vi "prop_value_pair_main.vi"(10 "Value Pair Properties In":T1={"X Value Pairs"={"Data Array"=[], "Show ticks"=TRUE, "Show grid lines"=TRUE, "Labels"=enum."Name"}, "Y Value Pairs"={"Data Array"=[], "Show ticks"=TRUE, "Show grid lines"=TRUE, "Labels"=enum."Value"}, "Z Value Pairs"={"Data Array"=[], "Show ticks"=TRUE, "Show grid lines"=TRUE, "Labels"=enum."Value"}}) -> (2 "Value Pair Properties Out":T1={"X Value Pairs"={"Data Array"=[], "Show ticks"=TRUE, "Show grid lines"=TRUE, "Labels"=enum."Name"}, "Y Value Pairs"={"Data Array"=[], "Show ticks"=TRUE, "Show grid lines"=TRUE, "Labels"=enum."Value"}, "Z Value Pairs"={"Data Array"=[], "Show ticks"=TRUE, "Show grid lines"=TRUE, "Labels"=enum."Value"}})   [LabVIEW 2020, in "3DPC_SurfacePlot.xctl"]
uses:
  <vilib>/Native 3D Graph/xcontrol/3DPC_SurfacePlot.xctl
  <vilib>/Native 3D Graph/typedefs/prop_value_pair_all.ctl
  <vilib>/Native 3D Graph/typedefs/prop_value_pair_1d.ctl
  <vilib>/Utility/miscctls.llb/LVPointTypeDef.ctl
panel:
  in  "Axis Select":u16(ring) caption="Axis" items=["X", "Y", "Z"]
  in  "done":refnum<user-event>
  in  "quit":refnum<user-event>
  in  "Axes Control Tab":enum32{"X", "Y", "Z"}(tab)
  in  "Labels X":u16(ring) caption="Labels" items=["Value", "None", "Name"]
  in  "Show Ticks X":bool
  in  "Show Grid Lines X":bool
  in  "Delete X":bool
  in  "Add X":bool
  in  "Pair Table X":i32(listbox)
  in  "Name X":string caption="Name"
  in  "Value X":dbl caption="Value"
  in  "Labels Y":u16(ring) caption="Labels" items=["Value", "None", "Name"]
  in  "Show Ticks Y":bool
  in  "Show Grid Lines Y":bool
  in  "Pair Table Y":i32(listbox)
  in  "Name Y":string caption="Name"
  in  "Value Y":dbl caption="Value"
  in  "Add Y":bool
  in  "Delete Y":bool
  in  "Labels Z":u16(ring) caption="Labels" items=["Value", "None", "Name"]
  in  "Show Ticks Z":bool
  in  "Show Grid Lines Z":bool
  in  "Pair Table Z":i32(listbox)
  in  "Name Z":string caption="Name"
  in  "Value Z":dbl caption="Value"
  in  "Delete Z":bool
  in  "Add Z":bool
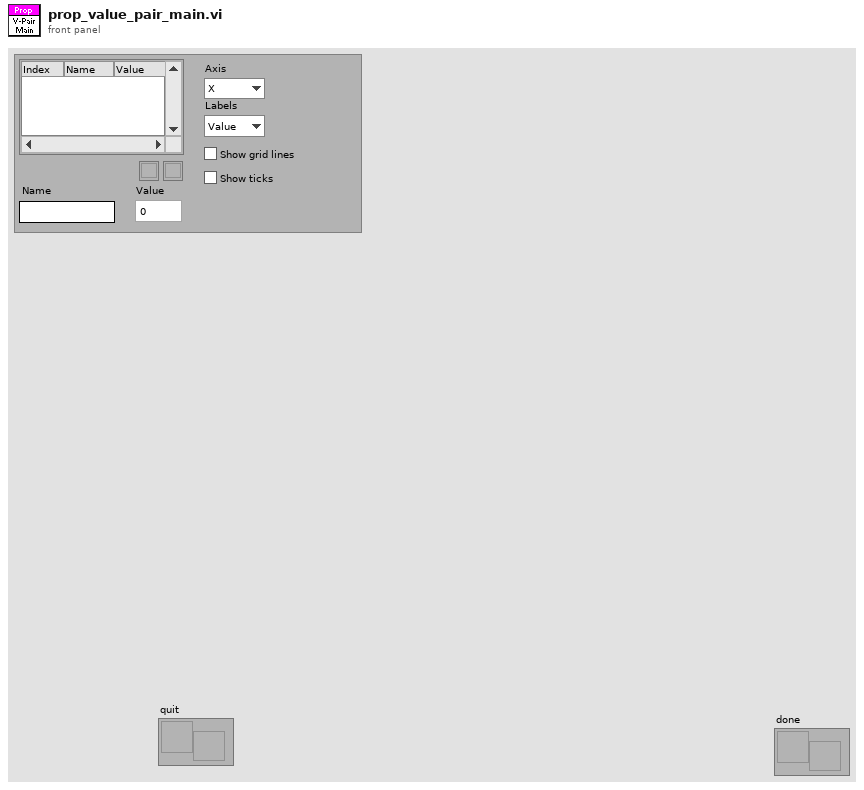
[diagram p1: front panel]
types:
  T1 = typedef "3DPC_SurfacePlot.xctl/prop_value_pair_all.ctl" = cluster{"X Value Pairs":cluster{"Data Array":cluster{"Value":sgl, "Index":i32, "Name":string}[], "Show ticks":bool, "Show grid lines":bool, "Labels":enum16{"Value", "None", "Name"}}, "Y Value Pairs":T2, "Z Value Pairs":T2}
  T2 = typedef "3DPC_SurfacePlot.xctl/prop_value_pair_1d.ctl" = cluster{"Data Array":cluster{"Value":sgl, "Index":i32, "Name":string}[], "Show ticks":bool, "Show grid lines":bool, "Labels":enum16{"Value", "None", "Name"}}
  T3 = typedef "LVPointTypeDef.ctl" = cluster{"Horizontal":i16, "Vertical":i16}
  T4 = cluster{"Value":sgl, "Index":i32, "Name":string}[]
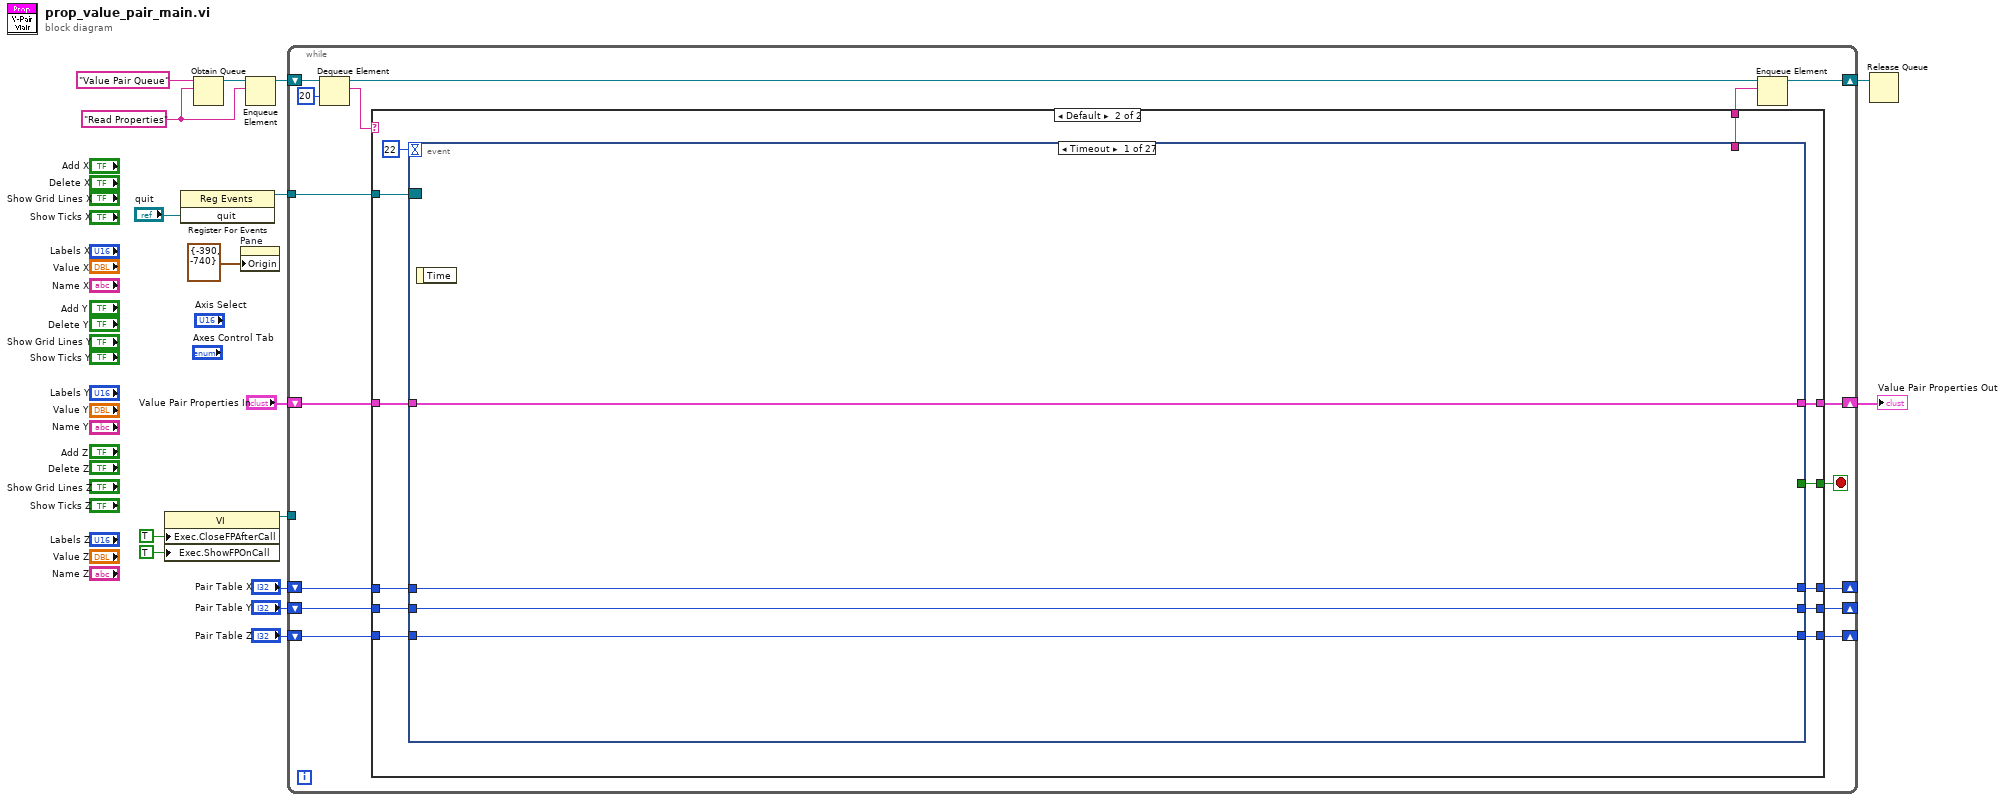
[diagram p0: block diagram]
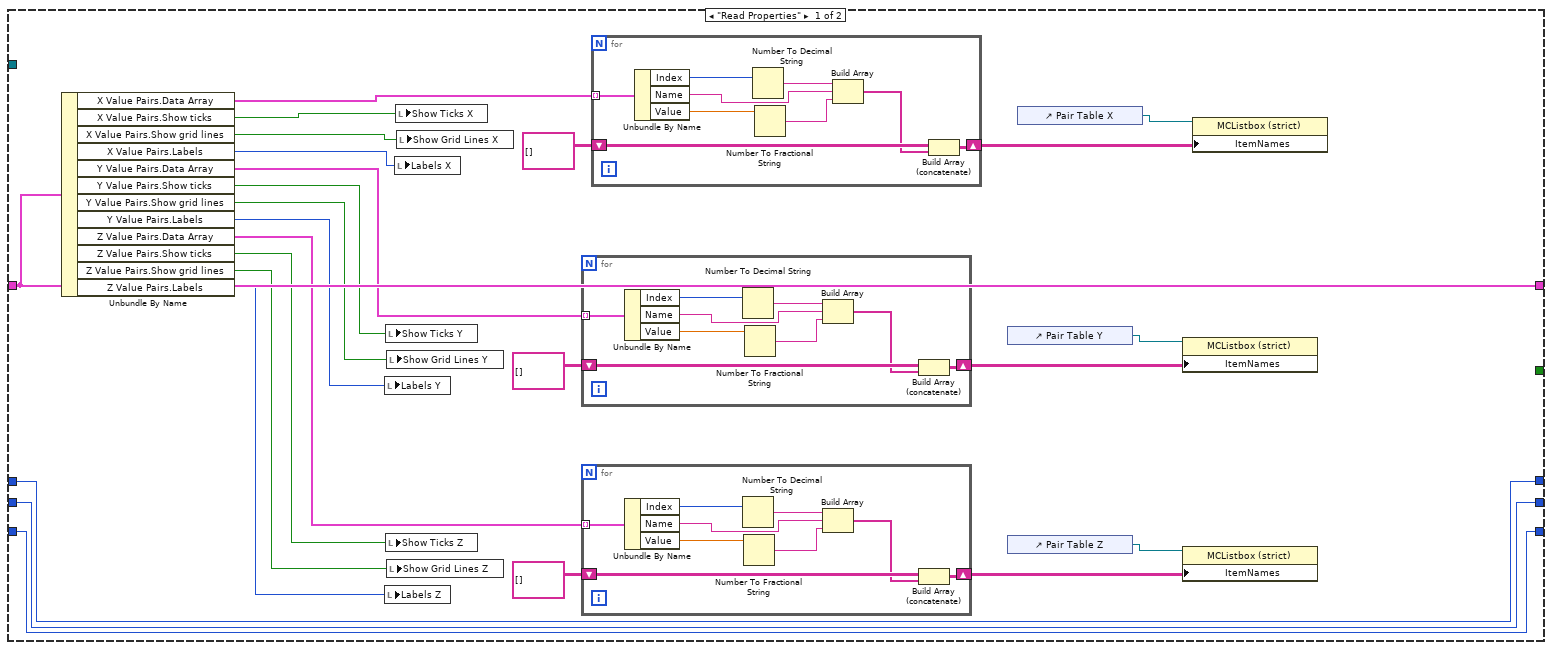
[diagram p2: hidden frame]
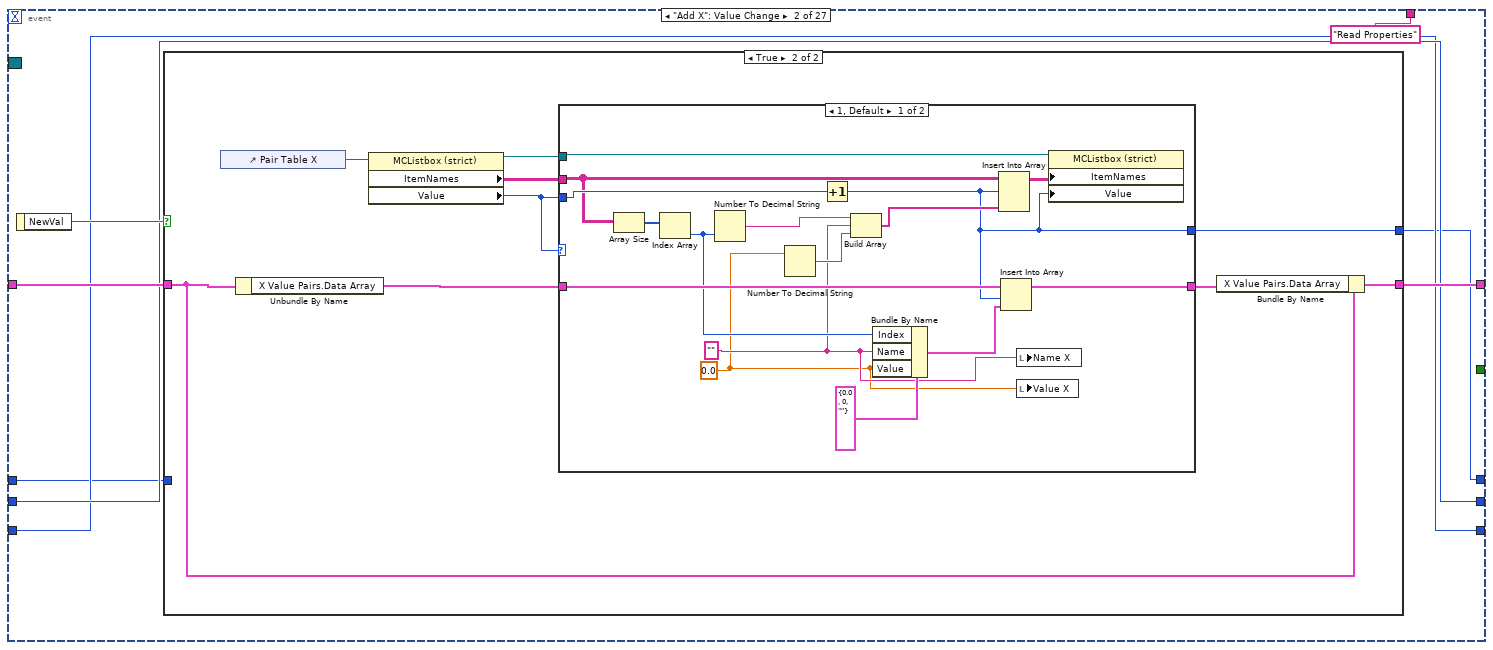
[diagram p3: hidden frame]
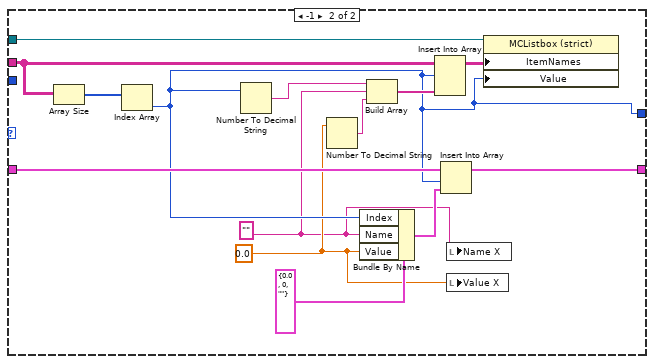
[diagram p5: hidden frame]
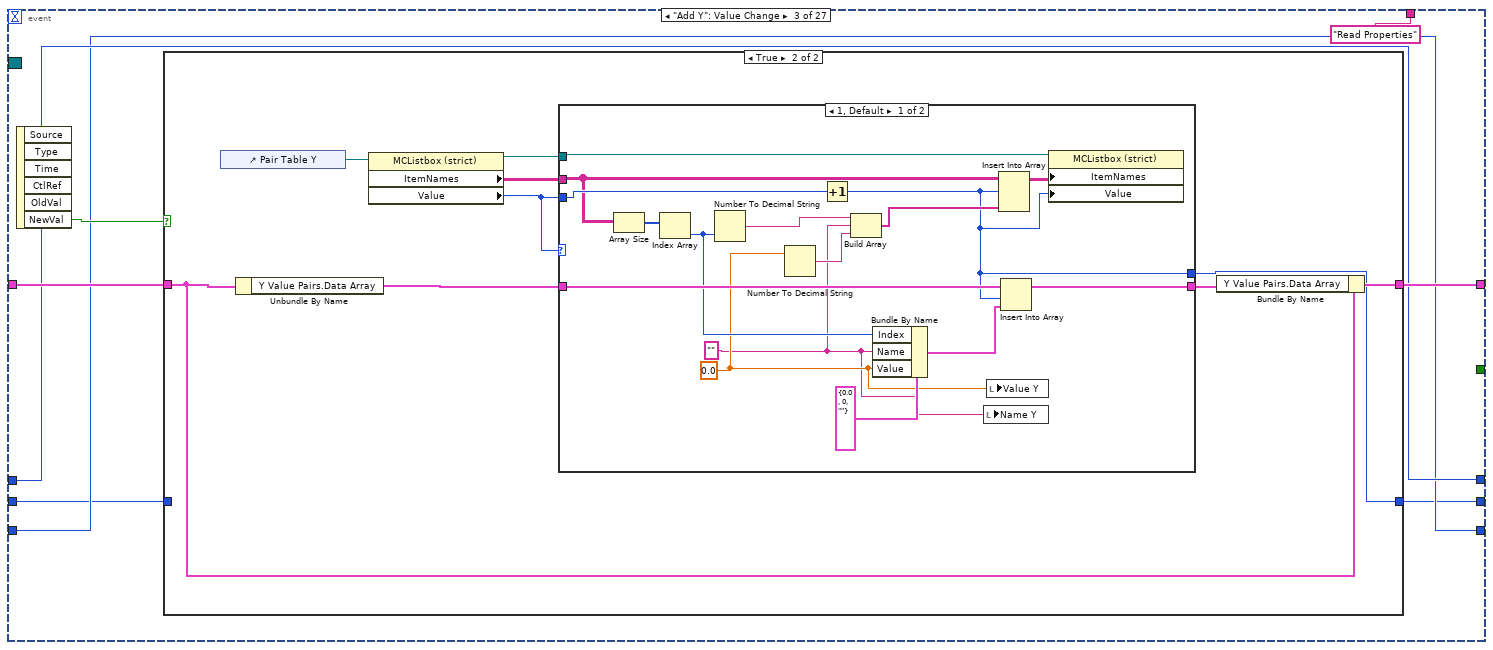
[diagram p6: hidden frame]
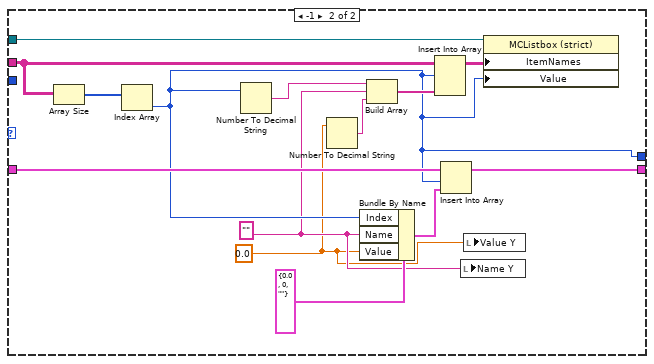
[diagram p8: hidden frame]
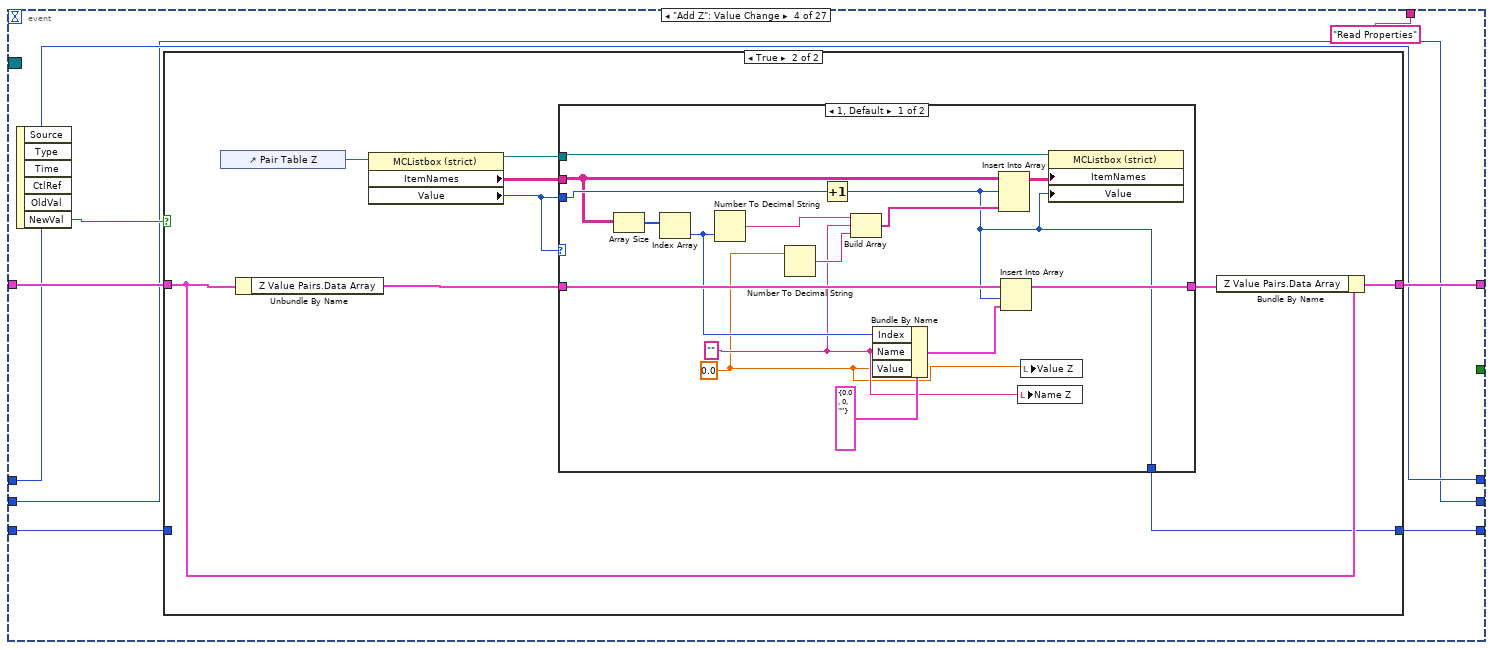
[diagram p9: hidden frame]
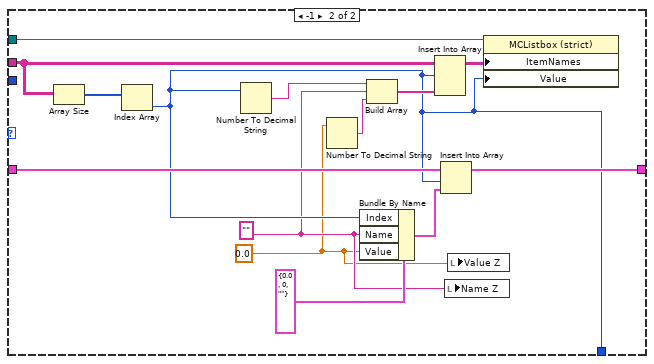
[diagram p11: hidden frame]
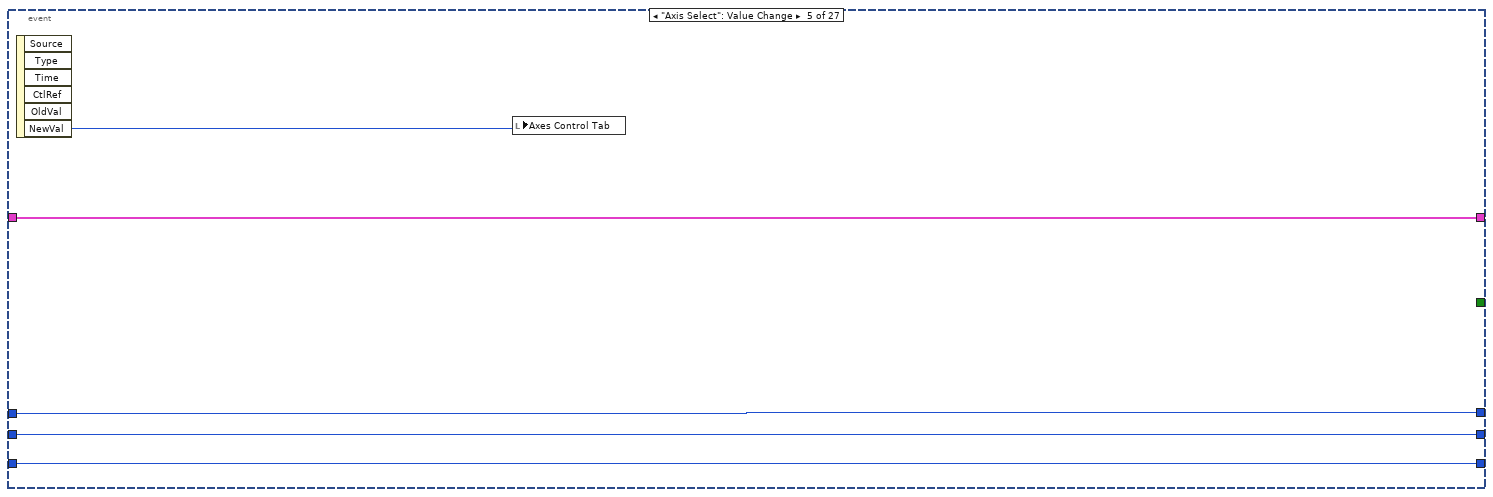
[diagram p12: hidden frame]
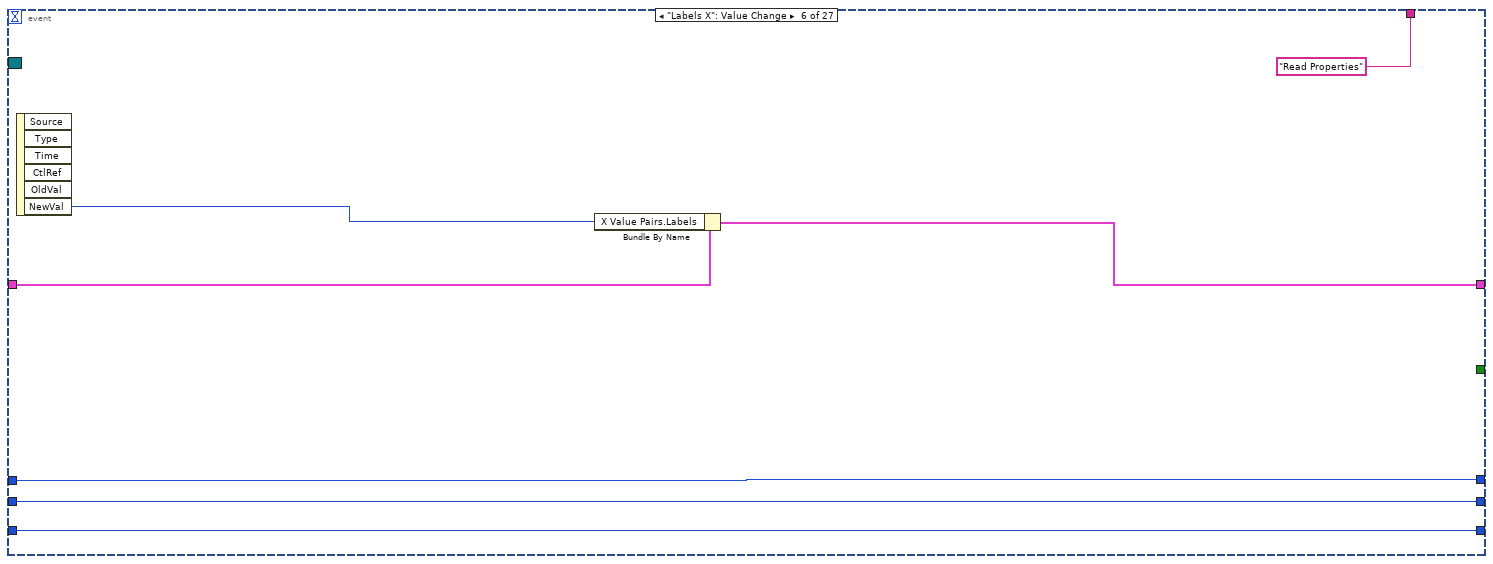
[diagram p13: hidden frame]
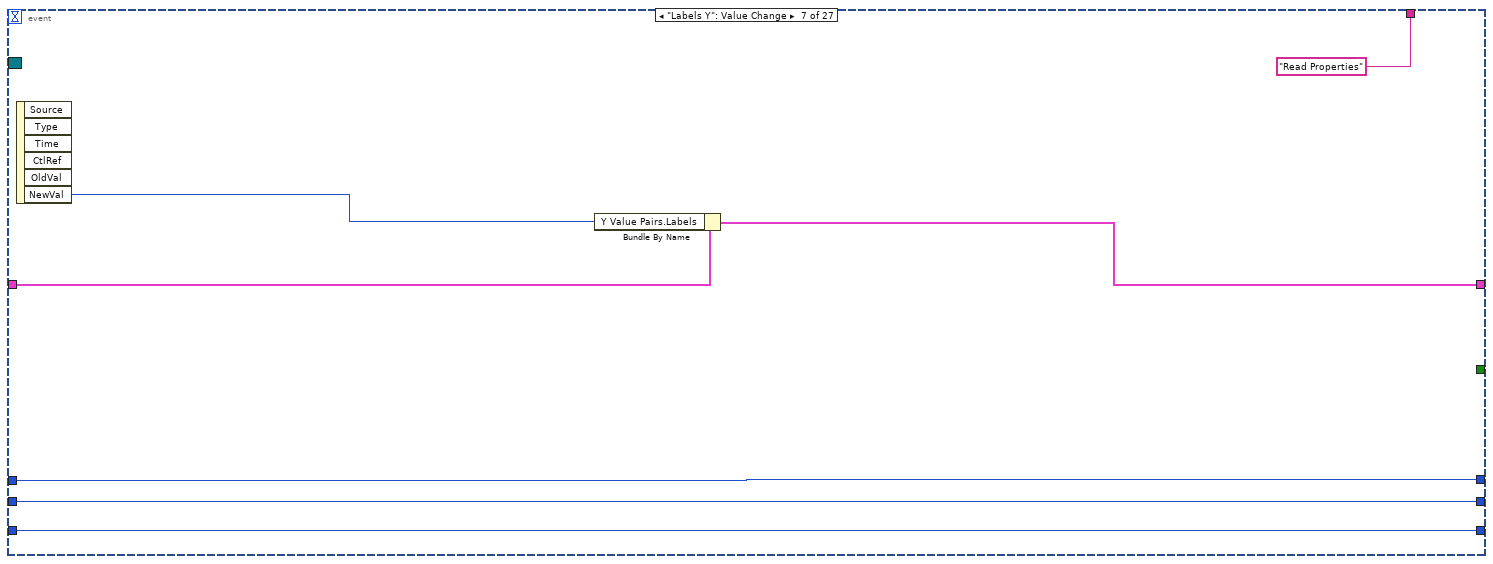
[diagram p14: hidden frame]
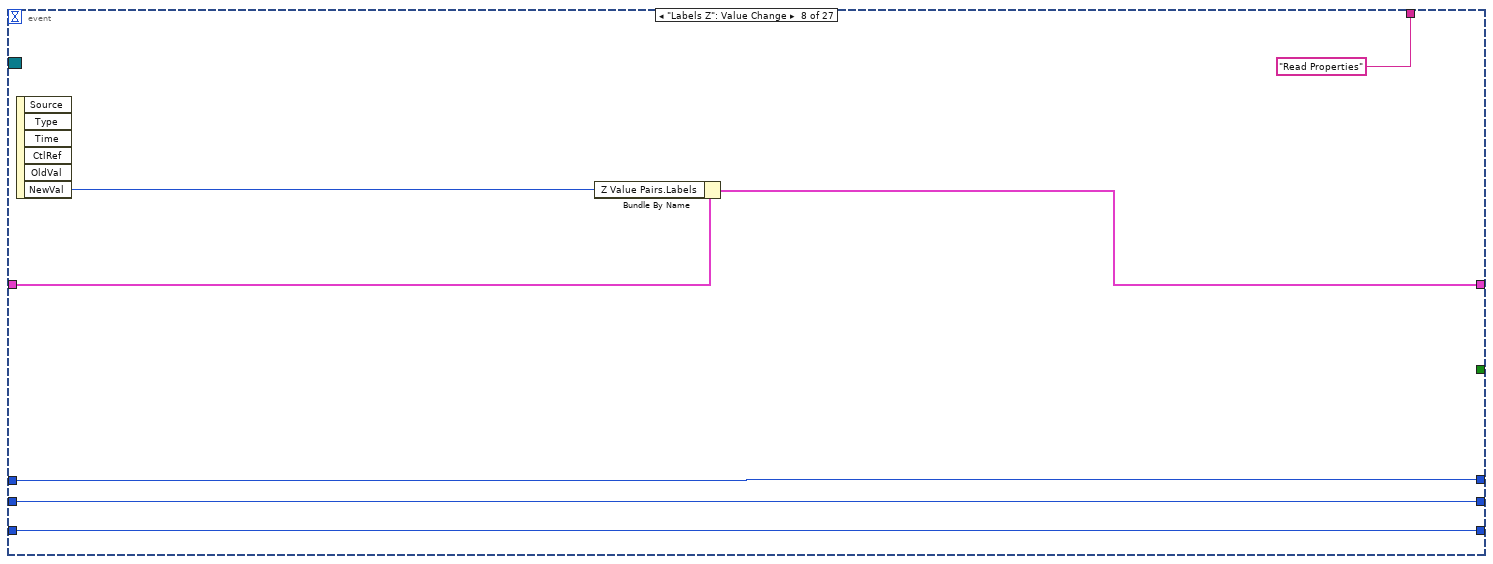
[diagram p15: hidden frame]
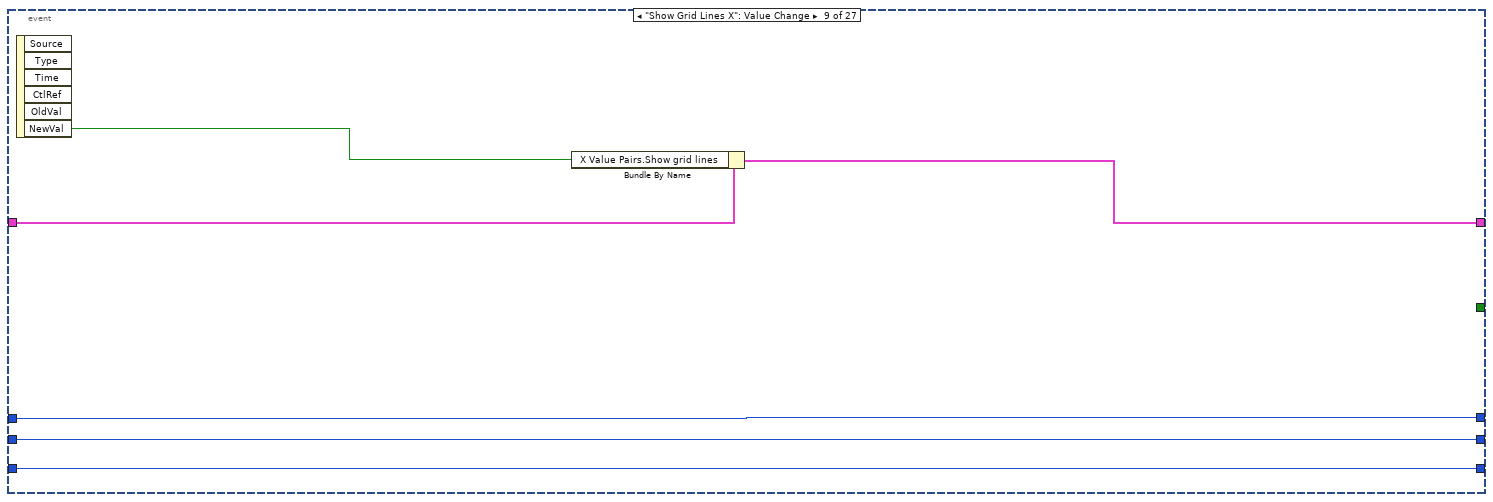
[diagram p16: hidden frame]
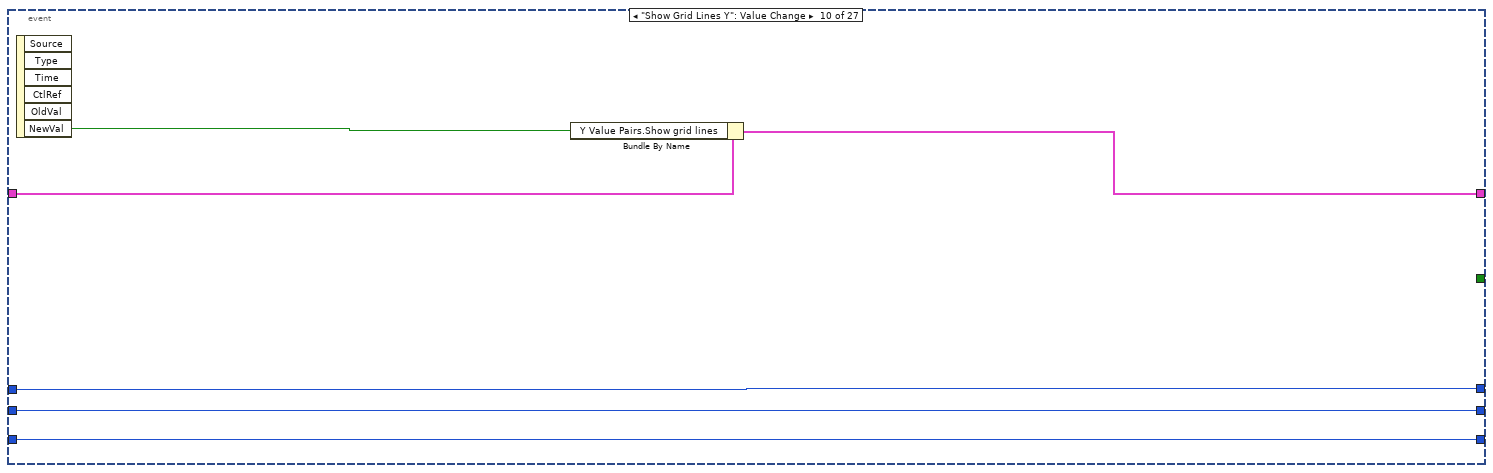
[diagram p17: hidden frame]
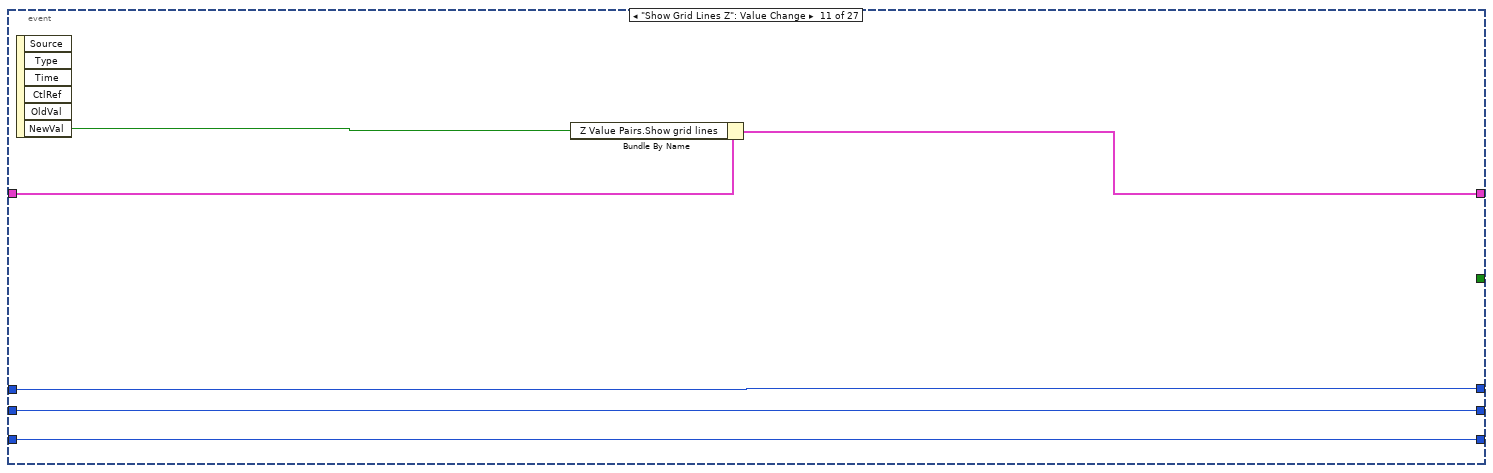
[diagram p18: hidden frame]
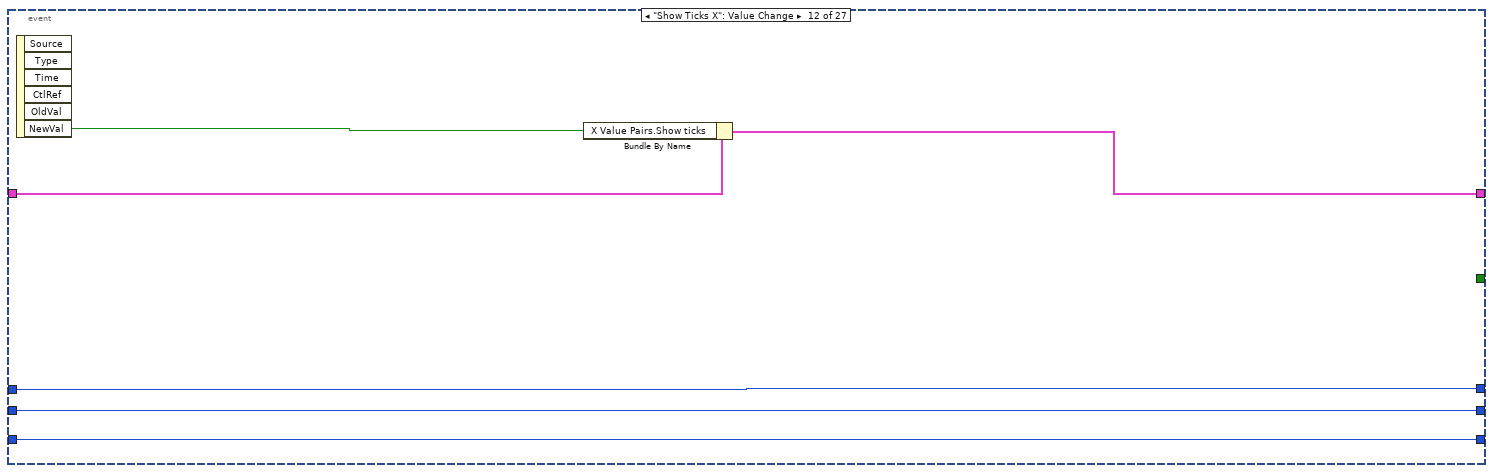
[diagram p19: hidden frame]
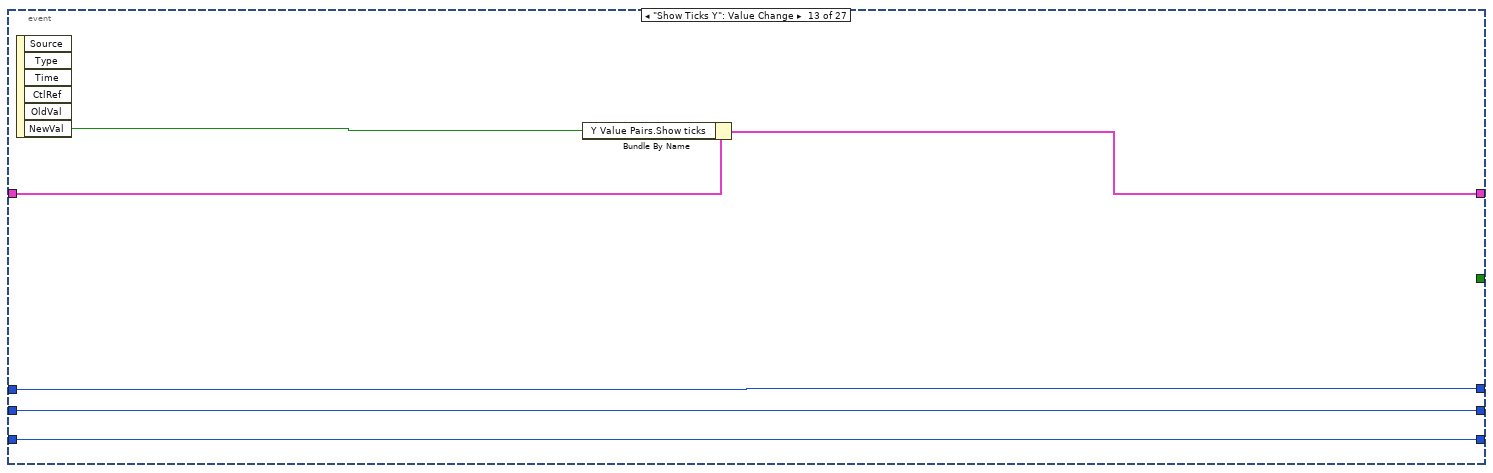
[diagram p20: hidden frame]
diagram:
  w13 = "Read Properties"
  n1 = property class="VI"("Exec.CloseFPAfterCall"=TRUE ("Execution:Close After Call"), "Exec.ShowFPOnCall"=TRUE ("Execution:Show Front Panel On Call")) -> (reference out=w10:refnum<vi>)  [unwired: 2 in, 1 out]
  n2 = register-events("quit") -> (reference out=w8:refnum<event-registration>)  [unwired: 2 in, 1 out]
  n3 = Obtain Queue(name (unnamed)="Value Pair Queue", element data type=w13) -> (queue out=w15:refnum<queue>)  [unwired: 3 in, 2 out]
  n4 = property on="Pane" class="Pane"("Origin"=T3 {"Horizontal"=-390, "Vertical"=-740}) -> ()  [unwired: 2 in, 2 out]
  n5 = Enqueue Element(queue=w15, element=w13) -> (queue out=w14:refnum<queue>)  [unwired: 1 in, 3 out]
  n6 = while {
    shift-right: [w29] -> w11
    shift-left: w14 -> [w32]
    shift-right: [w25] -> w12
    shift-left: "Value Pair Properties In" -> [w26]
    tunnel: w10 -> [_]
    tunnel: w8 -> [w23]
    shift-right: [w21] -> _
    shift-left: "Pair Table X" -> [w22]
    shift-right: [w20] -> _
    shift-left: "Pair Table Z" -> [w17]
    shift-right: [w19] -> _
    shift-left: "Pair Table Y" -> [w18]
    stop <- w24 stop-if-true
    n7 = Dequeue Element(queue=w32, timeout in ms (-1)=20) -> (queue out=w30:refnum<queue>, element=w31:string)  [unwired: 1 in, 2 out]
    n8 = case shown="Default" w31 {
      tunnel: [_ w95] -> w24
      tunnel: [_ w93] -> w28
      tunnel: w26 -> [w50 w96]
      tunnel: [w50 w94] -> w25
      tunnel: w23 -> [_ w91]
      tunnel: w22 -> [w35 w90]
      tunnel: w18 -> [w34 w89]
      tunnel: w17 -> [w33 w88]
      tunnel: [w35 w87] -> w21
      tunnel: [w33 w86] -> w20
      tunnel: [w34 w85] -> w19
      frame "Read Properties" {
        n9 = Unbundle By Name(w50) -> ("X Value Pairs.Data Array"=w57:T4, "X Value Pairs.Show ticks"=w55:bool, "X Value Pairs.Show grid lines"=w54:bool, "X Value Pairs.Labels"=w53:enum16{"Value", "None", "Name"}, "Y Value Pairs.Data Array"=w43:T4, "Y Value Pairs.Show ticks"=w42:bool, "Y Value Pairs.Show grid lines"=w41:bool, "Y Value Pairs.Labels"=w40:enum16{"Value", "None", "Name"}, "Z Value Pairs.Data Array"=w39:T4, "Z Value Pairs.Show ticks"=w38:bool, "Z Value Pairs.Show grid lines"=w37:bool, "Z Value Pairs.Labels"=w36:enum16{"Value", "None", "Name"})
        n10 = local write "Labels Y"(w40) -> ()
        n11 = local write "Labels Z"(w36) -> ()
        n12 = local write "Show Ticks Y"(w42) -> ()
        n13 = local write "Show Ticks Z"(w38) -> ()
        n14 = local write "Show Grid Lines Y"(w41) -> ()
        n15 = local write "Show Grid Lines Z"(w37) -> ()
        n16 = local write "Labels X"(w53) -> ()
        n17 = local write "Show Ticks X"(w55) -> ()
        n18 = local write "Show Grid Lines X"(w54) -> ()
        n19 = for {
          tunnel: w43 -> [w75] mode=indexing
          shift-right: [w70] -> w48
          shift-left: string[][] [] -> [w72]
          n20 = Unbundle By Name(w75) -> ("Index"=w74:i32, "Name"=w69:string, "Value"=w67:sgl)
          n21 = Number To Decimal String(number=w74) -> (decimal integer string=w73:string)  [unwired: 1 out]
          n22 = Number To Fractional String(number=w67) -> (F-format string=w68:string)  [unwired: 3 out]
          n23 = Build Array(w73, w69, w68) -> (w71:string[])
          n24 = Build Array (concatenate)(w72, w71) -> (w70:string[][])
        }
        n25 = for {
          tunnel: w39 -> [w66] mode=indexing
          shift-right: [w61] -> w45
          shift-left: string[][] [] -> [w63]
          n26 = Unbundle By Name(w66) -> ("Index"=w65:i32, "Name"=w60:string, "Value"=w58:sgl)
          n27 = Number To Decimal String(number=w65) -> (decimal integer string=w64:string)  [unwired: 1 out]
          n28 = Number To Fractional String(number=w58) -> (F-format string=w59:string)  [unwired: 3 out]
          n29 = Build Array(w64, w60, w59) -> (w62:string[])
          n30 = Build Array (concatenate)(w63, w62) -> (w61:string[][])
        }
        n31 = for {
          tunnel: w57 -> [w84] mode=indexing
          shift-right: [w79] -> w52
          shift-left: string[][] [] -> [w81]
          n32 = Unbundle By Name(w84) -> ("Index"=w83:i32, "Name"=w78:string, "Value"=w76:sgl)
          n33 = Number To Decimal String(number=w83) -> (decimal integer string=w82:string)  [unwired: 1 out]
          n34 = Number To Fractional String(number=w76) -> (F-format string=w77:string)  [unwired: 3 out]
          n35 = Build Array(w82, w78, w77) -> (w80:string[])
          n36 = Build Array (concatenate)(w81, w80) -> (w79:string[][])
        }
        n37 = control-ref of="Pair Table Y"() -> (w49:refnum<vi>)
        n38 = control-ref of="Pair Table Z"() -> (w44:refnum<vi>)
        n39 = control-ref of="Pair Table X"() -> (w51:refnum<vi>)
        n40 = property class="MCListbox (strict)"(reference=w49, "ItemNames"=w48) -> ()  [unwired: 1 in, 2 out]
        n41 = property class="MCListbox (strict)"(reference=w44, "ItemNames"=w45) -> ()  [unwired: 1 in, 2 out]
        n42 = property class="MCListbox (strict)"(reference=w51, "ItemNames"=w52) -> ()  [unwired: 1 in, 2 out]
      }
      frame Default {
        n43 = event shown="[0] Timeout" {
          selector: w91 -> [_ _ _ _ _ _ _ _ _ _ _ _ _ _ _ _ _ _ _ _ _ _ _ _ _ _ _]
          dyn-events: _ -> [_ _ _ _ _ _ _ _ _ _ _ _ _ _ _ _ _ _ _ _ _ _ _ _ _ _ _]
          timeout: 22 -> [_ _ _ _ _ _ _ _ _ _ _ _ _ _ _ _ _ _ _ _ _ _ _ _ _ _ _]
          tunnel: w96 -> [w100 w107 w156 w205 w251 w259 w266 w273 w279 w285 w291 w297 w303 w309 w317 w325 w333 w338 w354 w370 w392 w403 w414 w425 w432 w443 w455]
          tunnel: [_ _ _ _ _ _ _ _ _ _ _ _ _ _ _ _ _ _ _ _ _ _ _ _ TRUE _ FALSE ("NewVal")] -> w95
          tunnel: [w100 w106 w155 w204 w251 w257 w264 w271 w277 w283 w289 w295 w301 w307 w317 w325 w333 w337 w353 w369 w387 w398 w409 w420 w432 w438 w450] -> w94
          tunnel: [_ "Read Properties" "Read Properties" "Read Properties" _ "Read Properties" "Read Properties" "Read Properties" _ _ _ _ _ _ _ _ _ _ _ _ "Read Properties" "Read Properties" "Read Properties" "Read Properties" _ "Read Properties" "Read Properties"] -> w93
          tunnel: w90 -> [w99 w102 w154 w203 w250 w255 w262 w269 w276 w282 w288 w294 w300 w306 _ w318 w326 w334 w352 w366 w384 w395 w406 w417 w428 w433 w444]
          tunnel: w89 -> [w98 w105 w151 w202 w249 w254 w261 w268 w275 w281 w287 w293 w299 w305 w311 _ w327 w336 w350 w367 w383 w394 w405 w415 w427 w435 w445]
          tunnel: w88 -> [w97 w104 w153 w200 w248 w253 w260 w267 w274 w280 w286 w292 w298 w304 w310 w319 _ w335 w351 w368 w382 w393 w404 w416 w426 w434 w446]
          tunnel: [w99 w103 w154 w203 w250 w255 w262 w269 w276 w282 w288 w294 w300 w306 w312 w318 w326 w334 w352 w366 w384 w395 w406 w417 w428 w433 w444] -> w87
          tunnel: [w97 w104 w153 w201 w248 w253 w260 w267 w274 w280 w286 w292 w298 w304 w310 w319 w328 w335 w351 w368 w382 w393 w404 w416 w426 w434 w446] -> w86
          tunnel: [w98 w105 w152 w202 w249 w254 w261 w268 w275 w281 w287 w293 w299 w305 w311 w320 w327 w336 w350 w367 w383 w394 w405 w415 w427 w435 w445] -> w85
          event Timeout {
            n44 = event-data() -> ()  [unwired: 2 out]
          }
          event "Add X": Value Change {
            n45 = event-data() -> ("NewVal"=w108:bool)  [unwired: 1 out]
            n46 = case shown="True" w108 {
              tunnel: w107 -> [w110 w113]
              tunnel: [w110 w114] -> w106
              tunnel: [w109 w111] -> w103
              tunnel: w102 -> [w109 _]
              frame False {
              }
              frame True {
                n47 = control-ref of="Pair Table X"() -> (w119:refnum<vi>)
                n48 = Unbundle By Name(w113) -> ("X Value Pairs.Data Array"=w115:T4)
                n49 = property class="MCListbox (strict)"(reference=w119) -> (reference out=w118:refnum<vi>, "ItemNames"=w117:string[][], "Value"=w116:i32)  [unwired: 1 in, 1 out]
                n50 = case shown="1, Default" w116 {
                  tunnel: w118 -> [w135 w149]
                  tunnel: w117 -> [w130 w145]
                  tunnel: w116 -> [w131 _]
                  tunnel: w115 -> [w127 w140]
                  tunnel: [w123 w139] -> w112
                  tunnel: [w122 w138] -> w111
                  frame 1, Default {
                    w120 = sgl 0.0 ("Value")
                    w121 = "" ("decimal integer string")
                    n51 = Array Size(array=w130) -> (size(s)=w129:i32[])
                    n52 = Index Array(array=w129) -> (element=w125:i32)  [unwired: 1 in]
                    n53 = Number To Decimal String(number=w125) -> (decimal integer string=w132:string)  [unwired: 1 out]
                    n54 = Number To Decimal String(number=w120) -> (decimal integer string=w124:string)  [unwired: 1 out]
                    n55 = Increment(x=w131) -> (x+1=w122:i32)
                    n56 = Build Array(w132, w121, w124) -> (w133:string[])
                    n57 = Bundle By Name(cluster=cluster{"Value":sgl, "Index":i32, "Name":string} {"Value"=0.0, "Index"=0, "Name"=""}, "Index"=w125, "Name"=w121, "Value"=w120) -> (w126:cluster{"Value":sgl, "Index":i32, "Name":string})
                    n58 = Insert Into Array(array=w130, index (row)=w122, new element=w133) -> (w134:string[][])  [unwired: 1 in]
                    n59 = Insert Into Array(array=w127, index=w122, new element=w126) -> (w123:T4)
                    n60 = local write "Name X"(w121) -> ()
                    n61 = local write "Value X"(w120) -> ()
                    n62 = property class="MCListbox (strict)"(reference=w135, "ItemNames"=w134, "Value"=w122) -> ()  [unwired: 1 in, 2 out]
                  }
                  frame -1 {
                    w137 = sgl 0.0 ("Value")
                    w136 = "" ("decimal integer string")
                    n63 = Array Size(array=w145) -> (size(s)=w144:i32[])
                    n64 = Index Array(array=w144) -> (element=w138:i32)  [unwired: 1 in]
                    n65 = Number To Decimal String(number=w138) -> (decimal integer string=w146:string)  [unwired: 1 out]
                    n66 = Number To Decimal String(number=w137) -> (decimal integer string=w141:string)  [unwired: 1 out]
                    n67 = Bundle By Name(cluster=cluster{"Value":sgl, "Index":i32, "Name":string} {"Value"=0.0, "Index"=0, "Name"=""}, "Index"=w138, "Name"=w136, "Value"=w137) -> (w142:cluster{"Value":sgl, "Index":i32, "Name":string})
                    n68 = Build Array(w146, w136, w141) -> (w147:string[])
                    n69 = Insert Into Array(array=w145, index (row)=w138, new element=w147) -> (w148:string[][])  [unwired: 1 in]
                    n70 = Insert Into Array(array=w140, index=w138, new element=w142) -> (w139:T4)
                    n71 = local write "Name X"(w136) -> ()
                    n72 = local write "Value X"(w137) -> ()
                    n73 = property class="MCListbox (strict)"(reference=w149, "ItemNames"=w148, "Value"=w138) -> ()  [unwired: 1 in, 2 out]
                  }
                }
                n74 = Bundle By Name(cluster=w113, "X Value Pairs.Data Array"=w112) -> (w114:T1)
              }
            }
          }
          event "Add Y": Value Change {
            n75 = event-data() -> ("NewVal"=w157:bool)  [unwired: 6 out]
            n76 = case shown="True" w157 {
              tunnel: w156 -> [w159 w162]
              tunnel: [w159 w163] -> w155
              tunnel: [w158 w160] -> w152
              tunnel: w151 -> [w158 _]
              frame False {
              }
              frame True {
                n77 = control-ref of="Pair Table Y"() -> (w168:refnum<vi>)
                n78 = Unbundle By Name(w162) -> ("Y Value Pairs.Data Array"=w164:T4)
                n79 = property class="MCListbox (strict)"(reference=w168) -> (reference out=w167:refnum<vi>, "ItemNames"=w166:string[][], "Value"=w165:i32)  [unwired: 1 in, 1 out]
                n80 = case shown="1, Default" w165 {
                  tunnel: w167 -> [w184 w198]
                  tunnel: w166 -> [w179 w194]
                  tunnel: w165 -> [w180 _]
                  tunnel: w164 -> [w176 w189]
                  tunnel: [w172 w188] -> w161
                  tunnel: [w171 w187] -> w160
                  frame 1, Default {
                    w170 = sgl 0.0 ("Value")
                    w169 = "" ("decimal integer string")
                    n81 = Array Size(array=w179) -> (size(s)=w178:i32[])
                    n82 = Index Array(array=w178) -> (element=w174:i32)  [unwired: 1 in]
                    n83 = Number To Decimal String(number=w174) -> (decimal integer string=w181:string)  [unwired: 1 out]
                    n84 = Number To Decimal String(number=w170) -> (decimal integer string=w173:string)  [unwired: 1 out]
                    n85 = Increment(x=w180) -> (x+1=w171:i32)
                    n86 = Build Array(w181, w169, w173) -> (w182:string[])
                    n87 = Bundle By Name(cluster=cluster{"Value":sgl, "Index":i32, "Name":string} {"Value"=0.0, "Index"=0, "Name"=""}, "Index"=w174, "Name"=w169, "Value"=w170) -> (w175:cluster{"Value":sgl, "Index":i32, "Name":string})
                    n88 = local write "Name Y"(w169) -> ()
                    n89 = local write "Value Y"(w170) -> ()
                    n90 = Insert Into Array(array=w179, index (row)=w171, new element=w182) -> (w183:string[][])  [unwired: 1 in]
                    n91 = Insert Into Array(array=w176, index=w171, new element=w175) -> (w172:T4)
                    n92 = property class="MCListbox (strict)"(reference=w184, "ItemNames"=w183, "Value"=w171) -> ()  [unwired: 1 in, 2 out]
                  }
                  frame -1 {
                    w185 = sgl 0.0 ("Value")
                    w186 = "" ("decimal integer string")
                    n93 = Array Size(array=w194) -> (size(s)=w193:i32[])
                    n94 = Index Array(array=w193) -> (element=w187:i32)  [unwired: 1 in]
                    n95 = Number To Decimal String(number=w187) -> (decimal integer string=w195:string)  [unwired: 1 out]
                    n96 = Number To Decimal String(number=w185) -> (decimal integer string=w190:string)  [unwired: 1 out]
                    n97 = Bundle By Name(cluster=cluster{"Value":sgl, "Index":i32, "Name":string} {"Value"=0.0, "Index"=0, "Name"=""}, "Index"=w187, "Name"=w186, "Value"=w185) -> (w191:cluster{"Value":sgl, "Index":i32, "Name":string})
                    n98 = Build Array(w195, w186, w190) -> (w196:string[])
                    n99 = Insert Into Array(array=w194, index (row)=w187, new element=w196) -> (w197:string[][])  [unwired: 1 in]
                    n100 = Insert Into Array(array=w189, index=w187, new element=w191) -> (w188:T4)
                    n101 = local write "Name Y"(w186) -> ()
                    n102 = local write "Value Y"(w185) -> ()
                    n103 = property class="MCListbox (strict)"(reference=w198, "ItemNames"=w197, "Value"=w187) -> ()  [unwired: 1 in, 2 out]
                  }
                }
                n104 = Bundle By Name(cluster=w162, "Y Value Pairs.Data Array"=w161) -> (w163:T1)
              }
            }
          }
          event "Add Z": Value Change {
            n105 = event-data() -> ("NewVal"=w206:bool)  [unwired: 6 out]
            n106 = case shown="True" w206 {
              tunnel: w205 -> [w208 w211]
              tunnel: [w208 w212] -> w204
              tunnel: [w207 w209] -> w201
              tunnel: w200 -> [w207 _]
              frame False {
              }
              frame True {
                n107 = control-ref of="Pair Table Z"() -> (w217:refnum<vi>)
                n108 = Unbundle By Name(w211) -> ("Z Value Pairs.Data Array"=w213:T4)
                n109 = property class="MCListbox (strict)"(reference=w217) -> (reference out=w216:refnum<vi>, "ItemNames"=w215:string[][], "Value"=w214:i32)  [unwired: 1 in, 1 out]
                n110 = case shown="1, Default" w214 {
                  tunnel: w216 -> [w233 w247]
                  tunnel: w215 -> [w228 w243]
                  tunnel: w214 -> [w229 _]
                  tunnel: w213 -> [w225 w238]
                  tunnel: [w221 w237] -> w210
                  tunnel: [w220 w236] -> w209
                  frame 1, Default {
                    w218 = sgl 0.0 ("Value")
                    w219 = "" ("decimal integer string")
                    n111 = Array Size(array=w228) -> (size(s)=w227:i32[])
                    n112 = Index Array(array=w227) -> (element=w223:i32)  [unwired: 1 in]
                    n113 = Number To Decimal String(number=w223) -> (decimal integer string=w230:string)  [unwired: 1 out]
                    n114 = Number To Decimal String(number=w218) -> (decimal integer string=w222:string)  [unwired: 1 out]
                    n115 = Increment(x=w229) -> (x+1=w220:i32)
                    n116 = Build Array(w230, w219, w222) -> (w231:string[])
                    n117 = Bundle By Name(cluster=cluster{"Value":sgl, "Index":i32, "Name":string} {"Value"=0.0, "Index"=0, "Name"=""}, "Index"=w223, "Name"=w219, "Value"=w218) -> (w224:cluster{"Value":sgl, "Index":i32, "Name":string})
                    n118 = Insert Into Array(array=w228, index (row)=w220, new element=w231) -> (w232:string[][])  [unwired: 1 in]
                    n119 = Insert Into Array(array=w225, index=w220, new element=w224) -> (w221:T4)
                    n120 = local write "Name Z"(w219) -> ()
                    n121 = local write "Value Z"(w218) -> ()
                    n122 = property class="MCListbox (strict)"(reference=w233, "ItemNames"=w232, "Value"=w220) -> ()  [unwired: 1 in, 2 out]
                  }
                  frame -1 {
                    w234 = sgl 0.0 ("Value")
                    w235 = "" ("decimal integer string")
                    n123 = Array Size(array=w243) -> (size(s)=w242:i32[])
                    n124 = Index Array(array=w242) -> (element=w236:i32)  [unwired: 1 in]
                    n125 = Number To Decimal String(number=w236) -> (decimal integer string=w244:string)  [unwired: 1 out]
                    n126 = Number To Decimal String(number=w234) -> (decimal integer string=w239:string)  [unwired: 1 out]
                    n127 = Bundle By Name(cluster=cluster{"Value":sgl, "Index":i32, "Name":string} {"Value"=0.0, "Index"=0, "Name"=""}, "Index"=w236, "Name"=w235, "Value"=w234) -> (w240:cluster{"Value":sgl, "Index":i32, "Name":string})
                    n128 = Build Array(w244, w235, w239) -> (w245:string[])
                    n129 = Insert Into Array(array=w243, index (row)=w236, new element=w245) -> (w246:string[][])  [unwired: 1 in]
                    n130 = Insert Into Array(array=w238, index=w236, new element=w240) -> (w237:T4)
                    n131 = local write "Name Z"(w235) -> ()
                    n132 = local write "Value Z"(w234) -> ()
                    n133 = property class="MCListbox (strict)"(reference=w247, "ItemNames"=w246, "Value"=w236) -> ()  [unwired: 1 in, 2 out]
                  }
                }
                n134 = Bundle By Name(cluster=w211, "Z Value Pairs.Data Array"=w210) -> (w212:T1)
              }
            }
          }
          event "Axis Select": Value Change {
            n135 = event-data() -> ("NewVal"=w252:u16)  [unwired: 6 out]
            n136 = local write "Axes Control Tab"(w252) -> ()
          }
          event "Labels X": Value Change {
            n137 = event-data() -> ("NewVal"=w258:u16)  [unwired: 6 out]
            n138 = Bundle By Name(cluster=w259, "X Value Pairs.Labels"=w258) -> (w257:T1)
          }
          event "Labels Y": Value Change {
            n139 = event-data() -> ("NewVal"=w265:u16)  [unwired: 6 out]
            n140 = Bundle By Name(cluster=w266, "Y Value Pairs.Labels"=w265) -> (w264:T1)
          }
          event "Labels Z": Value Change {
            n141 = event-data() -> ("NewVal"=w272:u16)  [unwired: 6 out]
            n142 = Bundle By Name(cluster=w273, "Z Value Pairs.Labels"=w272) -> (w271:T1)
          }
          event "Show Grid Lines X": Value Change {
            n143 = event-data() -> ("NewVal"=w278:bool)  [unwired: 6 out]
            n144 = Bundle By Name(cluster=w279, "X Value Pairs.Show grid lines"=w278) -> (w277:T1)
          }
          event "Show Grid Lines Y": Value Change {
            n145 = event-data() -> ("NewVal"=w284:bool)  [unwired: 6 out]
            n146 = Bundle By Name(cluster=w285, "Y Value Pairs.Show grid lines"=w284) -> (w283:T1)
          }
          event "Show Grid Lines Z": Value Change {
            n147 = event-data() -> ("NewVal"=w290:bool)  [unwired: 6 out]
            n148 = Bundle By Name(cluster=w291, "Z Value Pairs.Show grid lines"=w290) -> (w289:T1)
          }
          event "Show Ticks X": Value Change {
            n149 = event-data() -> ("NewVal"=w296:bool)  [unwired: 6 out]
            n150 = Bundle By Name(cluster=w297, "X Value Pairs.Show ticks"=w296) -> (w295:T1)
          }
          event "Show Ticks Y": Value Change {
            n151 = event-data() -> ("NewVal"=w302:bool)  [unwired: 6 out]
            n152 = Bundle By Name(cluster=w303, "Y Value Pairs.Show ticks"=w302) -> (w301:T1)
          }
          event "Show Ticks Z": Value Change {
            n153 = event-data() -> ("NewVal"=w308:bool)  [unwired: 6 out]
            n154 = Bundle By Name(cluster=w309, "Z Value Pairs.Show ticks"=w308) -> (w307:T1)
          }
          event "Pair Table X": Value Change {
            n155 = event-data() -> ("NewVal"=w312:i32)  [unwired: 6 out]
            n156 = Unbundle By Name(w317) -> ("X Value Pairs.Data Array"=w316:T4)
            n157 = Index Array(array=w316, index=w312) -> (element=w315:cluster{"Value":sgl, "Index":i32, "Name":string})
            n158 = Unbundle By Name(w315) -> ("Value"=w314:sgl, "Name"=w313:string)
            n159 = local write "Name X"(w313) -> ()
            n160 = local write "Value X"(w314) -> ()
          }
          event "Pair Table Y": Value Change {
            n161 = event-data() -> ("NewVal"=w320:i32)  [unwired: 6 out]
            n162 = Unbundle By Name(w325) -> ("Y Value Pairs.Data Array"=w324:T4)
            n163 = Index Array(array=w324, index=w320) -> (element=w323:cluster{"Value":sgl, "Index":i32, "Name":string})
            n164 = Unbundle By Name(w323) -> ("Value"=w322:sgl, "Name"=w321:string)
            n165 = local write "Name Y"(w321) -> ()
            n166 = local write "Value Y"(w322) -> ()
          }
          event "Pair Table Z": Value Change {
            n167 = event-data() -> ("NewVal"=w328:i32)  [unwired: 6 out]
            n168 = Unbundle By Name(w333) -> ("Z Value Pairs.Data Array"=w332:T4)
            n169 = Index Array(array=w332, index=w328) -> (element=w331:cluster{"Value":sgl, "Index":i32, "Name":string})
            n170 = Unbundle By Name(w331) -> ("Value"=w330:sgl, "Name"=w329:string)
            n171 = local write "Name Z"(w329) -> ()
            n172 = local write "Value Z"(w330) -> ()
          }
          event "Delete X": Value Change {
            n173 = event-data() -> ("NewVal"=w339:bool)  [unwired: 6 out]
            n174 = case shown="True" w339 {
              tunnel: w338 -> [w340 w345]
              tunnel: [w340 w344] -> w337
              tunnel: w334 -> [_ w341]
              frame False {
              }
              frame True {
                n175 = Unbundle By Name(w345) -> ("X Value Pairs.Data Array"=w343:T4)
                n176 = control-ref of="Pair Table X"() -> (w349:refnum<vi>)
                n177 = property class="MCListbox (strict)"(reference=w349) -> (reference out=w347:refnum<vi>, "ItemNames"=w348:string[][])  [unwired: 1 in, 1 out]
                n178 = Delete From Array(array=w348, index (row)=w341) -> (array with subset deleted=w346:string[][])  [unwired: 2 in, 1 out]
                n179 = Delete From Array(array=w343, index=w341) -> (array with subset deleted=w342:T4)  [unwired: 1 in, 1 out]
                n180 = property class="MCListbox (strict)"(reference=w347, "ItemNames"=w346) -> ()  [unwired: 1 in, 2 out]
                n181 = Bundle By Name(cluster=w345, "X Value Pairs.Data Array"=w342) -> (w344:T1)
              }
            }
          }
          event "Delete Y": Value Change {
            n182 = event-data() -> ("NewVal"=w355:bool)  [unwired: 6 out]
            n183 = case shown="False" w355 {
              tunnel: w354 -> [w356 w361]
              tunnel: [w356 w360] -> w353
              tunnel: w350 -> [_ w357]
              frame False {
              }
              frame True {
                n184 = Unbundle By Name(w361) -> ("Y Value Pairs.Data Array"=w359:T4)
                n185 = control-ref of="Pair Table Y"() -> (w365:refnum<vi>)
                n186 = property class="MCListbox (strict)"(reference=w365) -> (reference out=w363:refnum<vi>, "ItemNames"=w364:string[][])  [unwired: 1 in, 1 out]
                n187 = Delete From Array(array=w364, index (row)=w357) -> (array with subset deleted=w362:string[][])  [unwired: 2 in, 1 out]
                n188 = Delete From Array(array=w359, index=w357) -> (array with subset deleted=w358:T4)  [unwired: 1 in, 1 out]
                n189 = property class="MCListbox (strict)"(reference=w363, "ItemNames"=w362) -> ()  [unwired: 1 in, 2 out]
                n190 = Bundle By Name(cluster=w361, "Y Value Pairs.Data Array"=w358) -> (w360:T1)
              }
            }
          }
          event "Delete Z": Value Change {
            n191 = event-data() -> ("NewVal"=w371:bool)  [unwired: 6 out]
            n192 = case shown="True" w371 {
              tunnel: w370 -> [w372 w377]
              tunnel: [w372 w376] -> w369
              tunnel: w368 -> [_ w373]
              frame False {
              }
              frame True {
                n193 = Unbundle By Name(w377) -> ("Z Value Pairs.Data Array"=w375:T4)
                n194 = control-ref of="Pair Table Z"() -> (w381:refnum<vi>)
                n195 = property class="MCListbox (strict)"(reference=w381) -> (reference out=w379:refnum<vi>, "ItemNames"=w380:string[][])  [unwired: 1 in, 1 out]
                n196 = Delete From Array(array=w380, index (row)=w373) -> (array with subset deleted=w378:string[][])  [unwired: 2 in, 1 out]
                n197 = Delete From Array(array=w375, index=w373) -> (array with subset deleted=w374:T4)  [unwired: 1 in, 1 out]
                n198 = property class="MCListbox (strict)"(reference=w379, "ItemNames"=w378) -> ()  [unwired: 1 in, 2 out]
                n199 = Bundle By Name(cluster=w377, "Z Value Pairs.Data Array"=w374) -> (w376:T1)
              }
            }
          }
          event "Value X": Value Change {
            n200 = event-data() -> ("NewVal"=w385:dbl)  [unwired: 6 out]
            n201 = Unbundle By Name(w392) -> ("X Value Pairs.Data Array"=w390:T4)
            n202 = Index Array(array=w390, index=w384) -> (element=w391:cluster{"Value":sgl, "Index":i32, "Name":string})
            n203 = Bundle By Name(cluster=w391, "Value"=w385) -> (w389:cluster{"Value":sgl, "Index":i32, "Name":string})
            n204 = Replace Array Subset(array=w390, new element=w389, index=w384) -> (w388:T4)
            n205 = Bundle By Name(cluster=w392, "X Value Pairs.Data Array"=w388) -> (w387:T1)
          }
          event "Value Y": Value Change {
            n206 = event-data() -> ("NewVal"=w396:dbl)  [unwired: 6 out]
            n207 = Unbundle By Name(w403) -> ("Y Value Pairs.Data Array"=w401:T4)
            n208 = Index Array(array=w401, index=w394) -> (element=w402:cluster{"Value":sgl, "Index":i32, "Name":string})
            n209 = Bundle By Name(cluster=w402, "Value"=w396) -> (w400:cluster{"Value":sgl, "Index":i32, "Name":string})
            n210 = Replace Array Subset(array=w401, new element=w400, index=w394) -> (w399:T4)
            n211 = Bundle By Name(cluster=w403, "Y Value Pairs.Data Array"=w399) -> (w398:T1)
          }
          event "Value Z": Value Change {
            n212 = event-data() -> ("NewVal"=w407:dbl)  [unwired: 6 out]
            n213 = Unbundle By Name(w414) -> ("Z Value Pairs.Data Array"=w412:T4)
            n214 = Index Array(array=w412, index=w404) -> (element=w413:cluster{"Value":sgl, "Index":i32, "Name":string})
            n215 = Bundle By Name(cluster=w413, "Value"=w407) -> (w411:cluster{"Value":sgl, "Index":i32, "Name":string})
            n216 = Replace Array Subset(array=w412, new element=w411, index=w404) -> (w410:T4)
            n217 = Bundle By Name(cluster=w414, "Z Value Pairs.Data Array"=w410) -> (w409:T1)
          }
          event "Name X": Value Change {
            n218 = event-data() -> ("NewVal"=w419:string)  [unwired: 6 out]
            n219 = Unbundle By Name(w425) -> ("X Value Pairs.Data Array"=w423:T4)
            n220 = Index Array(array=w423, index=w417) -> (element=w424:cluster{"Value":sgl, "Index":i32, "Name":string})
            n221 = Bundle By Name(cluster=w424, "Name"=w419) -> (w422:cluster{"Value":sgl, "Index":i32, "Name":string})
            n222 = Replace Array Subset(array=w423, new element=w422, index=w417) -> (w421:T4)
            n223 = Bundle By Name(cluster=w425, "X Value Pairs.Data Array"=w421) -> (w420:T1)
          }
          event User Event {
            n224 = event-data() -> ()  [unwired: 6 out]
            n225 = control-ref of="This VI"() -> (w430:refnum<vi>)
            n226 = Generate User Event(user event="done", event data cluster=w430) -> ()  [unwired: 2 in, 2 out]
          }
          event "Name Y": Value Change {
            n227 = event-data() -> ("NewVal"=w437:string)  [unwired: 6 out]
            n228 = Unbundle By Name(w443) -> ("Y Value Pairs.Data Array"=w441:T4)
            n229 = Index Array(array=w441, index=w435) -> (element=w442:cluster{"Value":sgl, "Index":i32, "Name":string})
            n230 = Bundle By Name(cluster=w442, "Name"=w437) -> (w440:cluster{"Value":sgl, "Index":i32, "Name":string})
            n231 = Replace Array Subset(array=w441, new element=w440, index=w435) -> (w439:T4)
            n232 = Bundle By Name(cluster=w443, "Y Value Pairs.Data Array"=w439) -> (w438:T1)
          }
          event "Name Z": Value Change {
            n233 = event-data() -> ("NewVal"=w449:string)  [unwired: 6 out]
            n234 = Unbundle By Name(w455) -> ("Z Value Pairs.Data Array"=w453:T4)
            n235 = Index Array(array=w453, index=w446) -> (element=w454:cluster{"Value":sgl, "Index":i32, "Name":string})
            n236 = Bundle By Name(cluster=w454, "Name"=w449) -> (w452:cluster{"Value":sgl, "Index":i32, "Name":string})
            n237 = Replace Array Subset(array=w453, new element=w452, index=w446) -> (w451:T4)
            n238 = Bundle By Name(cluster=w455, "Z Value Pairs.Data Array"=w451) -> (w450:T1)
          }
        }
      }
    }
    n239 = Enqueue Element(queue=w30, element=w28) -> (queue out=w29:refnum<queue>)  [unwired: 1 in, 3 out]
  }
  "Value Pair Properties Out" <- w12
  n240 = Release Queue(queue=w11) -> ()  [unwired: 1 in, 4 out]
